vi "Start_FPGA_FIFOs.vi"(8 "error in (no error)":errorcluster, 11 "ClusterOut":T1) -> (0 "error out":errorcluster)   [LabVIEW 2018]
uses:
  Controls/HWCluster.ctl
  Controls/Clusts/FPGA_Config_Clust.ctl
  Controls/Enums/TargetNumber.ctl
  <vilib>/rvi/interface/common/niFpgaWaitOnOcc.vi
  <vilib>/Utility/error.llb/Error Cluster From Error Code.vi
  <vilib>/rvi/interface/nirviMethod/nirviMethod.xnode
  <vilib>/FPGAPlugInAG/Dynamic/niLvFpga_ConfigureFifo_Dynamic.vi
  <vilib>/rvi/errors/niLvFpgaMergeErrorWithErrorCode.vi
  <vilib>/FPGAPlugInAG/Dynamic/niLvFpga_StartFifo_Dynamic.vi
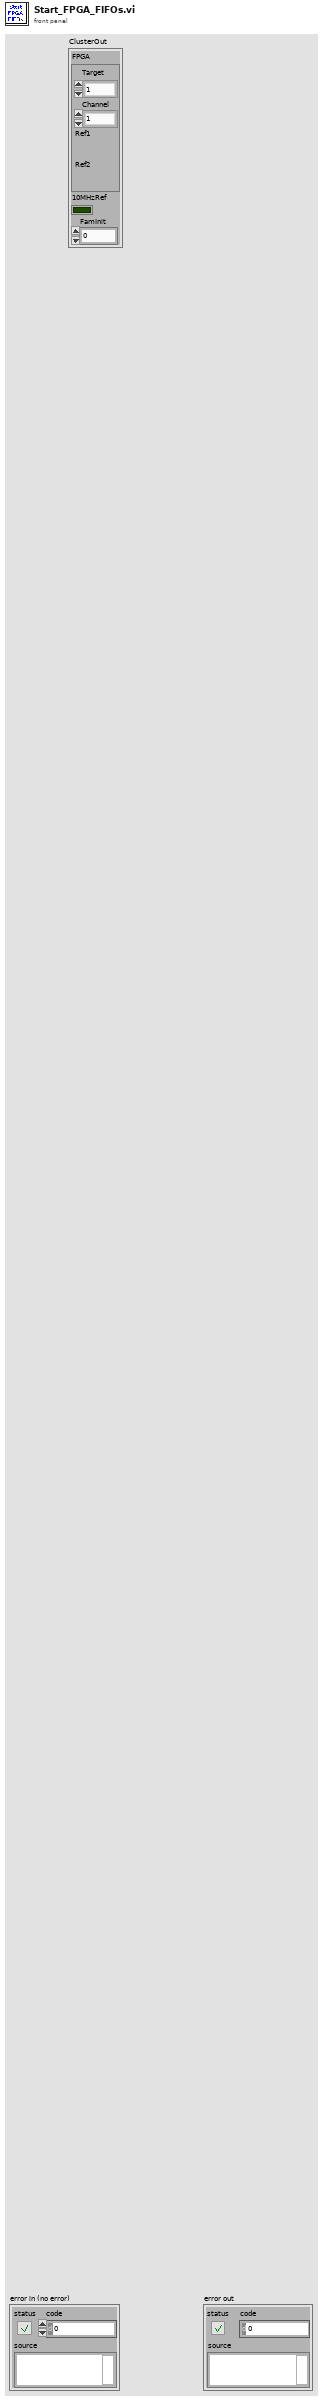
[diagram p1: front panel]
types:
  T1 = typedef "HWCluster.ctl" = cluster{"FPGA":T2, "10MHzRef":bool, "FamInit":i32}
  T2 = typedef "FPGA_Config_Clust.ctl" = cluster{"Target":T3, "Channel":T3, "Ref1":refnum<k20>, "Ref2":refnum<k20>}
  T3 = typedef "TargetNumber.ctl" = enum16{"1", "2", "3", "4"}
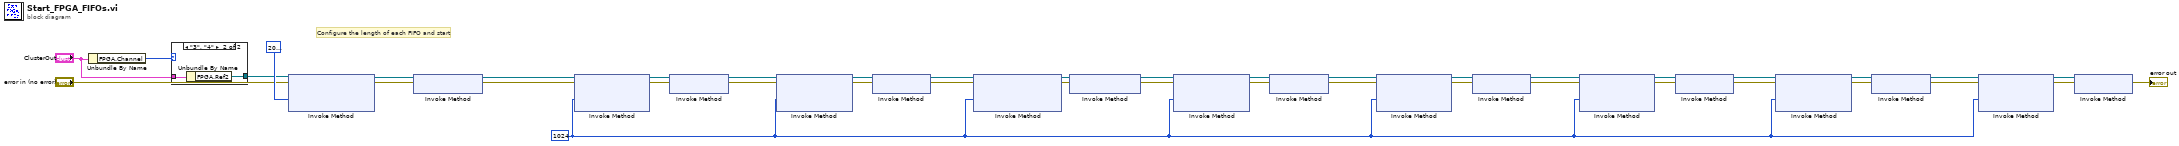
[diagram p0: block diagram]
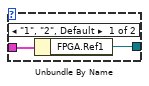
[diagram p2: hidden frame]
diagram:
  w1 = u32 1024 ("Requested Depth")
  # "Configure the length of each FIFO and start"
  n1 = Unbundle By Name("ClusterOut") -> ("FPGA.Channel"=w39:T3)
  n2 = case shown="\"3\", \"4\"" w39 {
    tunnel: "ClusterOut" -> [w43 w45]
    tunnel: [w42 w44] -> w37
    frame "1", "2", Default {
      n3 = Unbundle By Name(w43) -> ("FPGA.Ref1"=w42:refnum<k20>)
    }
    frame "3", "4" {
      n4 = Unbundle By Name(w45) -> ("FPGA.Ref2"=w44:refnum<k20>)
    }
  }
  n5 = xnode "Invoke Method"("FPGA VI Reference In"=w37, "error in"="error in (no error)", "Requested Depth"=u32 2000000 ("Num Samples")) -> ("FPGA VI Reference Out"=w36:refnum<k20>, "error out"=w35:errorcluster)  [unwired: 1 out]
  n6 = xnode "Invoke Method"("FPGA VI Reference In"=w36, "error in"=w35) -> ("FPGA VI Reference Out"=w32:refnum<k20>, "error out"=w31:errorcluster)
  n7 = xnode "Invoke Method"("FPGA VI Reference In"=w32, "error in"=w31, "Requested Depth"=w1) -> ("FPGA VI Reference Out"=w40:refnum<k20>, "error out"=w41:errorcluster)  [unwired: 1 out]
  n8 = xnode "Invoke Method"("FPGA VI Reference In"=w40, "error in"=w41) -> ("FPGA VI Reference Out"=w28:refnum<k20>, "error out"=w27:errorcluster)
  n9 = xnode "Invoke Method"("FPGA VI Reference In"=w28, "error in"=w27, "Requested Depth"=w1) -> ("FPGA VI Reference Out"=w30:refnum<k20>, "error out"=w29:errorcluster)  [unwired: 1 out]
  n10 = xnode "Invoke Method"("FPGA VI Reference In"=w30, "error in"=w29) -> ("FPGA VI Reference Out"=w5:refnum<k20>, "error out"=w2:errorcluster)
  n11 = xnode "Invoke Method"("FPGA VI Reference In"=w5, "error in"=w2, "Requested Depth"=w1) -> ("FPGA VI Reference Out"=w6:refnum<k20>, "error out"=w7:errorcluster)  [unwired: 1 out]
  n12 = xnode "Invoke Method"("FPGA VI Reference In"=w6, "error in"=w7) -> ("FPGA VI Reference Out"=w4:refnum<k20>, "error out"=w3:errorcluster)
  n13 = xnode "Invoke Method"("FPGA VI Reference In"=w4, "error in"=w3, "Requested Depth"=w1) -> ("FPGA VI Reference Out"=w22:refnum<k20>, "error out"=w21:errorcluster)  [unwired: 1 out]
  n14 = xnode "Invoke Method"("FPGA VI Reference In"=w22, "error in"=w21) -> ("FPGA VI Reference Out"=w25:refnum<k20>, "error out"=w26:errorcluster)
  n15 = xnode "Invoke Method"("FPGA VI Reference In"=w25, "error in"=w26, "Requested Depth"=w1) -> ("FPGA VI Reference Out"=w23:refnum<k20>, "error out"=w24:errorcluster)  [unwired: 1 out]
  n16 = xnode "Invoke Method"("FPGA VI Reference In"=w23, "error in"=w24) -> ("FPGA VI Reference Out"=w10:refnum<k20>, "error out"=w9:errorcluster)
  n17 = xnode "Invoke Method"("FPGA VI Reference In"=w10, "error in"=w9, "Requested Depth"=w1) -> ("FPGA VI Reference Out"=w11:refnum<k20>, "error out"=w12:errorcluster)  [unwired: 1 out]
  n18 = xnode "Invoke Method"("FPGA VI Reference In"=w11, "error in"=w12) -> ("FPGA VI Reference Out"=w19:refnum<k20>, "error out"=w20:errorcluster)
  n19 = xnode "Invoke Method"("FPGA VI Reference In"=w19, "error in"=w20, "Requested Depth"=w1) -> ("FPGA VI Reference Out"=w17:refnum<k20>, "error out"=w18:errorcluster)  [unwired: 1 out]
  n20 = xnode "Invoke Method"("FPGA VI Reference In"=w17, "error in"=w18) -> ("FPGA VI Reference Out"=w14:refnum<k20>, "error out"=w13:errorcluster)
  n21 = xnode "Invoke Method"("FPGA VI Reference In"=w14, "error in"=w13, "Requested Depth"=w1) -> ("FPGA VI Reference Out"=w16:refnum<k20>, "error out"=w15:errorcluster)  [unwired: 1 out]
  n22 = xnode "Invoke Method"("FPGA VI Reference In"=w16, "error in"=w15) -> ("error out"=→"error out":errorcluster)  [unwired: 1 out]
